vi "robotSimulation.vi"(10 "Config":T1 {"Motor"."Tf (Nm)" format="%#_13g"; "Motor"."KT (Nm/A)" format="%#_13g"; "Motor"."R (ohms)" format="%#_13g"; "Motor"."Ke (V)" format="%#_13g"}, 11 "Duty Cycle":dbl) -> (1 "Position":dbl, 2 "Velocity":dbl, 3 "Accel":dbl)   [LabVIEW 2017, in "Pure Pursuit.lvlib"]
uses:
  Pure Pursuit.lvlib
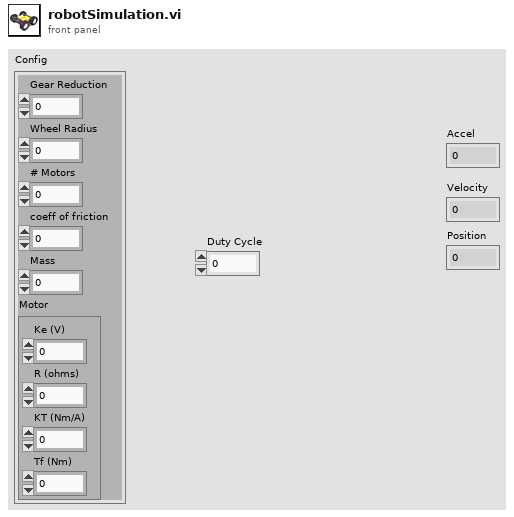
[diagram p1: front panel]
types:
  T1 = cluster{"Gear Reduction":dbl, "Wheel Radius":dbl, "# Motors":u32, "coeff of friction":dbl, "Mass":dbl, "Motor":cluster{"Ke (V)":dbl, "R (ohms)":dbl, "KT (Nm/A)":dbl, "Tf (Nm)":dbl}}
  T2 = cluster{"Ke (V)":dbl, "R (ohms)":dbl, "KT (Nm/A)":dbl, "Tf (Nm)":dbl}
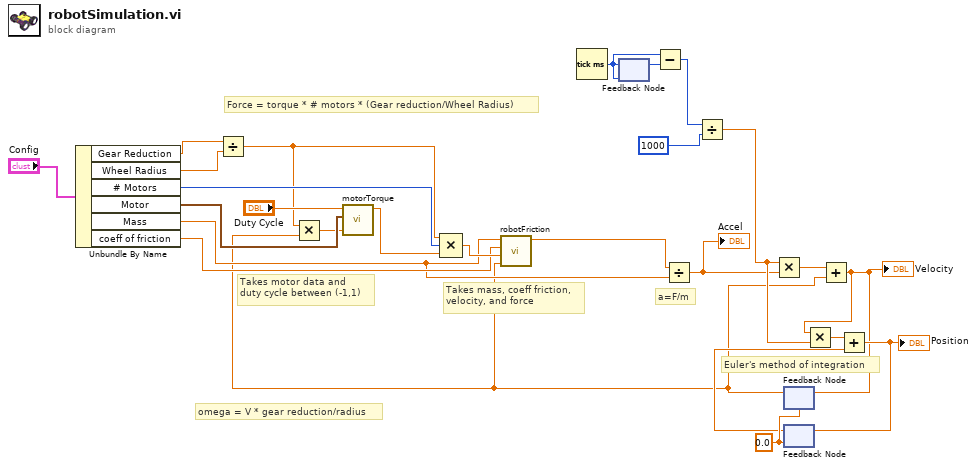
[diagram p0: block diagram]
diagram:
  w15 = 0.0
  # "omega = V * gear reduction/radius"
  # "Euler's method of integration"
  # "a=F/m"
  # "Force = torque * # motors * (Gear reduction/Wheel Radius)"
  # "Takes mass, coeff friction,\nvelocity, and force"
  # "Takes motor data and\nduty cycle between (-1,1)"
  n1 = Unbundle By Name("Config") -> ("Gear Reduction"=w22:dbl, "Wheel Radius"=w21:dbl, "# Motors"=w23:u32, "Motor"=w8:T2, "Mass"=w16:dbl, "coeff of friction"=w19:dbl)
  n2 = Divide(x=w22, y=w21) -> (x/y=w9:dbl)
  n3 = Tick Count (ms)() -> (millisecond timer value=w2:u32)
  n4 = feedback-in #1(w2) -> ()
  n5 = feedback #1(w2) -> (w3:u32)
  n6 = Subtract(x=w2, y=w3) -> (x-y=w1:u32)
  n7 = Divide(x=w1, y=u32 1000) -> (x/y=w11:dbl)
  n8 = feedback #2(w15) -> (w6:dbl)
  n9 = Multiply(x=w9, y=w6) -> (x*y=w7:dbl)
  n10 = call "motorTorque.vi"("omega"=w7, "Motor"=w8, "Duty Cycle"="Duty Cycle") -> ("Total Torque"=w24:dbl)  [unwired: 7 in]
  n11 = Compound Arithmetic op=MULTIPLY(w9, w23, w24) -> (w20:dbl)
  n12 = call "robotFriction.vi"("V in"=w6, "F in"=w20, "coeff friction"=w19, "Mass"=w16) -> ("Force out"=w17:dbl)  [unwired: 7 in]
  n13 = Divide(x=w17, y=w16) -> (x/y=w4:dbl)
  "Accel" <- w4
  n14 = Multiply(x=w11, y=w4) -> (x*y=w12:dbl)
  n15 = feedback #3(w15) -> (w13:dbl)
  n16 = Add(x=w12, y=w6) -> (x+y=w5:dbl)
  "Velocity" <- w5
  n17 = feedback-in #2(w5) -> ()
  n18 = Multiply(x=w5, y=w11) -> (x*y=w14:dbl)
  n19 = Add(x=w14, y=w13) -> (x+y=w10:dbl)
  "Position" <- w10
  n20 = feedback-in #3(w10) -> ()
